vi "Calibrate from file.vi"() -> ()   [LabVIEW 2015]
uses:
  <vilib>/measure/matone.llb/Extract Single Tone Information 1 Chan.vi
  <vilib>/measure/NI_MAPro.lvlib
panel:
  out "Sampling rate":dbl
  out "Calibrated range":dbl
  in  "Expected amplitude":dbl format="%#_6p"
  out "detected phase (deg)":dbl format="%.2p"
  out "detected amplitude":dbl format="%.2p"
  out "detected frequency":dbl format="%.2p"
  out "Waveform Graph":waveform(dbl)(graph)
  in  "Channel name":string="CH0"
  in  "File Path Control":path
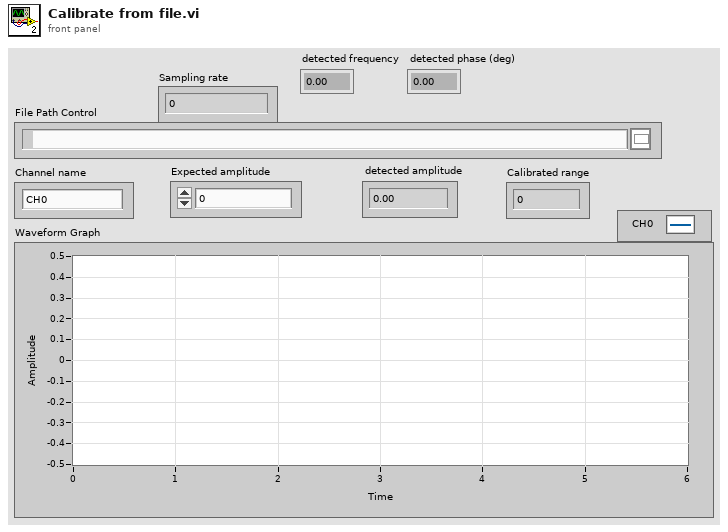
[diagram p1: front panel]
types:
  T1 = enum32{"none", "input signal", "detected signal", "residual signal"}
  T2 = enum16{"open", "open or create", "create or replace", "create", "open (read-only)"}
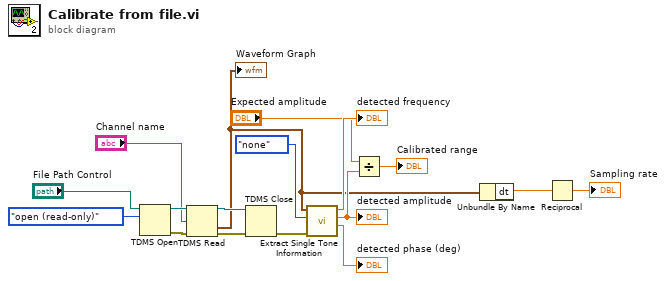
[diagram p0: block diagram]
diagram:
  n1 = TDMS Open(10:T2."open (read-only)" ("operation (0:open)"), 11:"File Path Control") -> (0:w14:errorcluster, 3:w15:refnum<k34>)  [unwired: 5 in]
  n2 = TDMS Read(0:w15, 7:"Channel name", 11:w14) -> (4:w11:refnum<k34>, 10:w3:waveform(dbl), 15:w12:errorcluster)  [unwired: 5 in, 3 out]
  "Waveform Graph" <- w3
  n3 = TDMS Close(8:w12, 11:w11) -> (0:w7:errorcluster)  [unwired: 1 out]
  n4 = call-poly <vilib>:"Extract Single Tone Information.vi"("error in (no error)"=w7, "export mode"=T1."none", "time signal in"=w3) -> ("detected phase (deg)"=→"detected phase (deg)":dbl, "detected amplitude"=w5:dbl, "detected frequency"=→"detected frequency":dbl)  [unwired: 3 in, 3 out]
  "detected amplitude" <- w5
  n5 = Divide(x="Expected amplitude", y=w5) -> (x/y=→"Calibrated range":dbl)
  n6 = Unbundle By Name(w3) -> ("dt"=w2:dbl)
  n7 = Reciprocal(x=w2) -> (1/x=→"Sampling rate":dbl)
